vi "Check if Time to Log.vi"(0 "Data Log Times IN":u32[](array[numeric]), 1 "Data Log Rate (ms)":u32, 2 "Pumps Present":bool[](array[boolean])=[FALSE, FALSE, FALSE, FALSE, FALSE, FALSE], 3 "AKLH Log Times IN":u32[][](array[numeric]), 4 "AKLH Rate (ms)":u32, 5 "In Spec":bool[](array[boolean])=[FALSE, FALSE, FALSE, FALSE, FALSE, FALSE], 6 "Test Profile":T2[](array[typedef]) {"Pump Cmds"."Pump 6\nCmd" min=0 format="%#.1f"; "Pump Cmds"."Pump 5\nCmd" min=0 format="%#.1f"; "Pump Cmds"."Pump 4\nCmd" min=0 format="%#.1f"; "Pump Cmds"."Pump 3\nCmd" min=0 format="%#.1f"; "Pump Cmds"."Pump 2\nCmd" min=0 format="%#.1f"; "Pump Cmds"."Pump 1\nCmd" min=0 format="%#.1f"; "Temp\nCmd" min=-60 max=100; "Pressure\nCmd" max=20; "PS\nCmd" min=0 max=20 format="%#.2f"; "Time (s)" min=0.0 format="%#.2g"}, 7 "Current Step":i32=2, 8 "Pump Data":T1={"Voltages"=[0.015201568603515625, 0.00335693359375, 0.003021240234375, 0.12260055541992188, 0.06085968017578125, 0.052234649658203125], "PumpCurrent"=[0.015201568603515625, 0.00335693359375, 0.003021240234375, 0.12260055541992188, 0.06085968017578125, 0.052234649658203125], "Speed"=[0.0, 0.0, 0.0, 0.0, 0.0, 0.0], "ControllerCurrent"=[0.015201568603515625, 0.00335693359375, 0.003021240234375, 0.12260055541992188, 0.06085968017578125, 0.052234649658203125], "Pressure"=[0.015201568603515625, 0.00335693359375, 0.003021240234375, 0.12260055541992188, 0.06085968017578125, 0.052234649658203125], "Flow"=[0.0, 0.0, 0.0, 0.125, 0.0625, 0.0625], "Elapsed Time (Display)"=[7.1, 7.1, 7.1, 458133.45, 458138.85000000003, 458126.75], "Avg Pressure"=0.0, "Avg Speed"=0.0, "Elapsed Time"=[4074.9003000000002, 4074.9003000000002, 4074.9003000000002, 4074.9003000000002, 4074.9003000000002, 4074.9003000000002], "Diagnostic"=[0.0, 0.0, 0.0, 0.0, 0.0, 0.0]} {"Diagnostic" format="%#.0f"; "Elapsed Time" format="%<%H:%M:%S>t"; "Elapsed Time (Display)" format="%<%H:%M:%S>t"; "Speed" format="%#_4f"; "ControllerCurrent" format="%#.1g"; "Pressure" format="%#.0f"; "Flow" format="%#.0f"; "PumpCurrent" format="%#.1g"; "Voltages" format="%#.0f"}, 9 "Step Time Left":dbl=0.21101045608520508, 11 "Target Speeds":u16[](array[numeric]), 13 "AKLH Filenames":string[](array[string])) -> (20 "Log Data":bool[](array[boolean]), 21 "Data Log Times OUT":u32[](array[numeric]), 22 "Log AKLH":bool[](array[boolean]), 23 "AKLH Log Times OUT":u32[][](array[numeric]), 24 "AKLH Filename":string, 25 "Target Speed":u16)   [LabVIEW 2019]
uses:
  Type Defs/Test Step.ctl
  Type Defs/Pump Cmds.ctl
  Controls/Pump Data.ctl
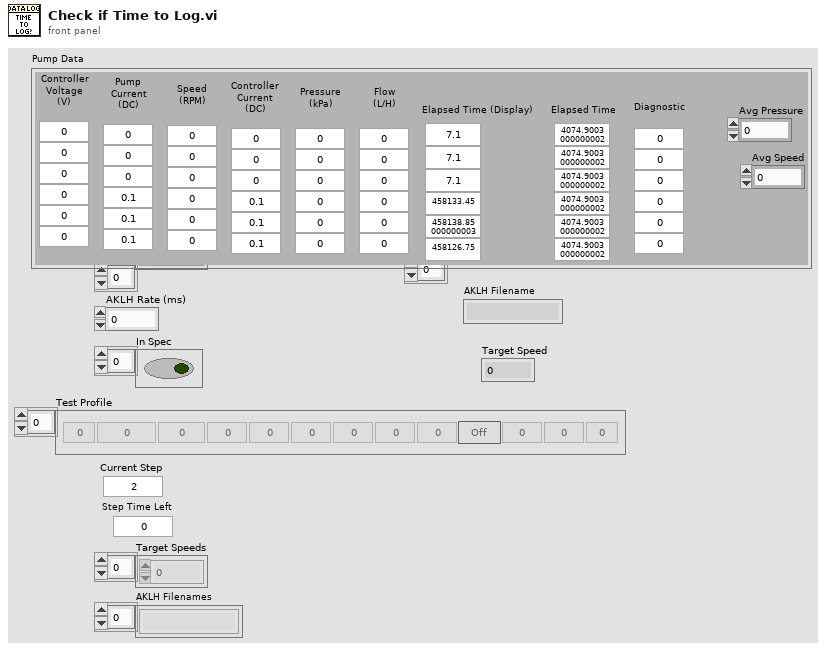
[diagram p1: front panel]
types:
  T1 = typedef "Pump Data.ctl" = cluster{"Voltages":dbl[], "PumpCurrent":dbl[], "Speed":dbl[], "ControllerCurrent":dbl[], "Pressure":dbl[], "Flow":dbl[], "Elapsed Time (Display)":dbl[], "Avg Pressure":dbl, "Avg Speed":dbl, "Elapsed Time":dbl[], "Diagnostic":dbl[]}
  T2 = typedef "Test Step.ctl" = cluster{"Step":u8, "Time (s)":dbl, "Target\nSpeed":u16, "Pump Cmds":T3, "Relays":bool, "PS\nCmd":sgl, "Pressure\nCmd":u16, "Temp\nCmd":i16}
  T3 = typedef "Pump Cmds.ctl" = cluster{"Pump 1\nCmd":sgl, "Pump 2\nCmd":sgl, "Pump 3\nCmd":sgl, "Pump 4\nCmd":sgl, "Pump 5\nCmd":sgl, "Pump 6\nCmd":sgl}
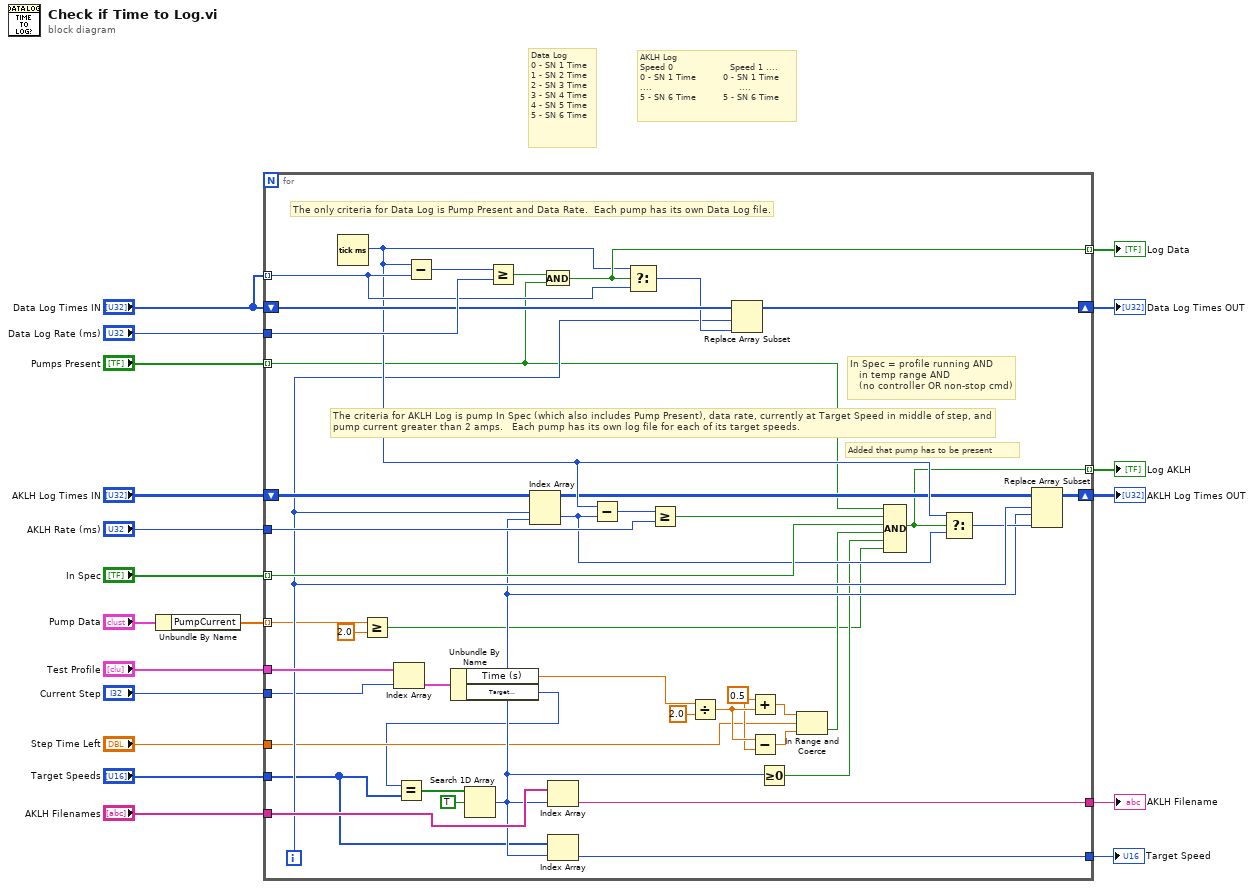
[diagram p0: block diagram]
diagram:
  # "AKLH Log\nSpeed 0                   Speed 1 ....\n0 - SN 1 Time         0 - SN 1 Time\n....                             ....\n5 - SN 6 Time         5 - SN 6 Time"
  # "Data Log\n0 - SN 1 Time\n1 - SN 2 Time\n2 - SN 3 Time\n3 - SN 4 Time\n4 - SN 5 Time\n5 - SN 6 Time"
  n1 = Unbundle By Name("Pump Data") -> ("PumpCurrent"=w1:dbl[])
  n2 = for {
    shift-right: [w56] -> w12
    shift-left: "Data Log Times IN" -> [w58]
    shift-right: [w41] -> w6
    shift-left: "AKLH Log Times IN" -> [w42]
    tunnel: "In Spec" -> [w45] mode=indexing
    tunnel: "Test Profile" -> [w54]
    tunnel: "Current Step" -> [w23]
    tunnel: "Step Time Left" -> [w30]
    tunnel: "Pumps Present" -> [w25] mode=indexing
    tunnel: "Data Log Times IN" -> [w59] mode=indexing
    tunnel: "Data Log Rate (ms)" -> [w61]
    tunnel: [w55] -> w11 mode=indexing
    tunnel: "Target Speeds" -> [w24]
    tunnel: "AKLH Filenames" -> [w50]
    tunnel: [w49] -> w8
    tunnel: "AKLH Rate (ms)" -> [w47]
    tunnel: [w38] -> w7 mode=indexing
    tunnel: [w37] -> w5
    tunnel: w1 -> [w28] mode=indexing
    i -> [w40]
    w33 = 0.5 ("y")
    # "In Spec = profile running AND\n   in temp range AND\n   (no controller OR non-stop cmd)"
    # "Added that pump has to be present"
    # "The criteria for AKLH Log is pump In Spec (which also includes Pump Present), data rate, currently at Target Speed in middle of step, and\npump current greater than 2 amps.   Each pump has its own log file for each of its target speeds."
    # "The only criteria for Data Log is Pump Present and Data Rate.  Each pump has its own Data Log file."
    n3 = Tick Count (ms)() -> (millisecond timer value=w44:u32)
    n4 = Greater Or Equal?(x=w28, y=2.0) -> (x >= y?=w26:bool)
    n5 = Index Array(array=w54, index=w23) -> (element=w22:T2)
    n6 = Subtract(x=w44, y=w59) -> (x-y=w62:u32)
    n7 = Unbundle By Name(w22) -> ("Time (s)"=w21:dbl, "Target\nSpeed"=w20:u16)
    n8 = Equal?(x=w20, y=w24) -> (x = y?=w52:bool[])
    n9 = Search 1D Array(1D array=w52, element=TRUE) -> (index of element=w36:i32)  [unwired: 1 in]
    n10 = Greater Or Equal?(x=w62, y=w61) -> (x >= y?=w60:bool)
    n11 = Index Array(array=w42, index (row)=w40, index (col)=w36) -> (element=w43:u32)
    n12 = And(x=w60, y=w25) -> (x .and. y?=w55:bool)
    n13 = Index Array(array=w50, index=w36) -> (element=w49:string)
    n14 = Index Array(array=w24, index=w36) -> (element=w37:u16)
    n15 = Subtract(x=w44, y=w43) -> (x-y=w48:u32)
    n16 = Select(t=w44, s=w55, f=w59) -> (s? t:f=w57:u32)
    n17 = Greater Or Equal?(x=w48, y=w47) -> (x >= y?=w46:bool)
    n18 = Divide(x=w21, y=2.0) -> (x/y=w34:dbl)
    n19 = Replace Array Subset(array=w58, new element=w57, index=w40) -> (w56:u32[])
    n20 = Add(x=w33, y=w34) -> (x+y=w32:dbl)
    n21 = Subtract(x=w34, y=w33) -> (x-y=w31:dbl)
    n22 = Greater Or Equal To 0?(x=w36) -> (x >= 0?=w35:bool)
    n23 = In Range and Coerce(upper limit=w32, x=w30, lower limit=w31) -> (In Range?=w29:bool)  [unwired: 1 out]
    n24 = Compound Arithmetic op=AND(w25, w46, w45, w29, w35, w26) -> (w38:bool)
    n25 = Select(t=w44, s=w38, f=w43) -> (s? t:f=w39:u32)
    n26 = Replace Array Subset(array=w42, new element=w39, index (row)=w40, index (col)=w36) -> (w41:u32[][])
  }
  "Data Log Times OUT" <- w12
  "Log Data" <- w11
  "AKLH Filename" <- w8
  "Log AKLH" <- w7
  "AKLH Log Times OUT" <- w6
  "Target Speed" <- w5
